vi "ProcessArray.vi"(4 "Plot Data":bool, 6 "Aquire Data":bool, 8 "File Path In":path, 11 "array in":sgl[][](array[numeric])) -> (0 "file path out":path, 1 "residue":dbl, 2 "intercept":dbl, 3 "Array out":T1(array[cluster]))   [LabVIEW 2019, in "SMU.lvclass"]
uses:
  SMU.lvclass
  <vilib>/Utility/file.llb/Write Delimited Spreadsheet (string).vi
  <vilib>/Utility/file.llb/Write Delimited Spreadsheet (DBL).vi
  <vilib>/Analysis/NI_AALPro.lvlib
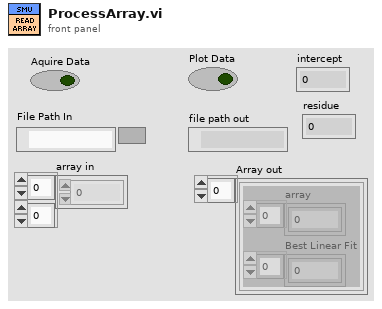
[diagram p1: front panel]
types:
  T1 = cluster{"array":sgl[], "Best Linear Fit":dbl[]}[]
  T2 = cluster{"array in":sgl[], "Best Linear Fit":dbl[]}
  T3 = cluster{"array in":sgl[], "Best Linear Fit":dbl[]}[]
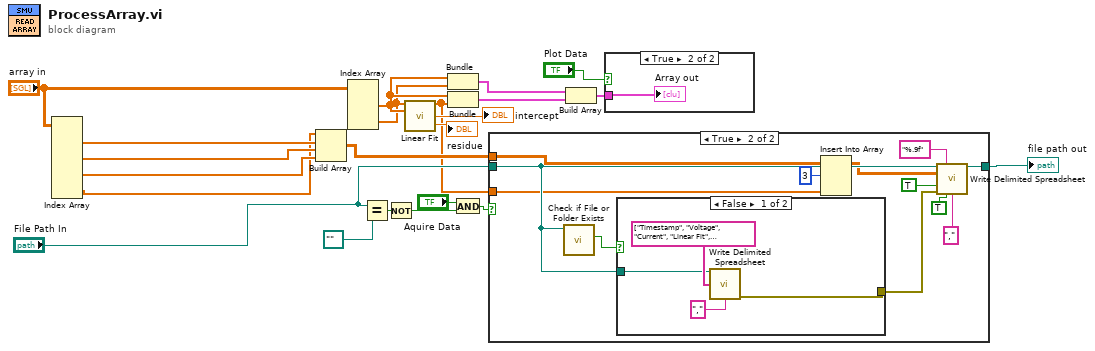
[diagram p0: block diagram]
diagram:
  n1 = Index Array(array="array in") -> (element #1=w6:sgl[], element #2=w2:sgl[], element #3=w5:sgl[], element #4=w1:sgl[])  [unwired: 8 in]
  n2 = Build Array(w1, w6, w2, w5) -> (w4:sgl[][])
  n3 = Index Array(array="array in") -> (element #1=w19:sgl[], element #2=w18:sgl[])  [unwired: 4 in]
  n4 = Equal?(x="File Path In", y=path "") -> (x = y?=w8:bool)
  n5 = Not(x=w8) -> (.not. x?=w20:bool)
  n6 = call <vilib>:"Linear Fit.vi"("Y"=w18, "X"=w19) -> ("Best Linear Fit"=w3:dbl[], "intercept"=→"intercept":dbl, "residue"=→"residue":dbl)  [unwired: 9 in, 2 out]
  n7 = Bundle("array in"=w19, "array in"=w18) -> (w16:cluster{"array in":sgl[], "array in":sgl[]})  [unwired: 1 in]
  n8 = Bundle("array in"=w19, "Best Linear Fit"=w3) -> (w17:T2)  [unwired: 1 in]
  n9 = And(x="Aquire Data", y=w20) -> (x .and. y?=w22:bool)
  n10 = case shown="True" w22 {
    tunnel: [w23 w35] -> w13
    tunnel: "File Path In" -> [w23 w31]
    tunnel: w4 -> [_ w28]
    tunnel: w3 -> [_ w25]
    frame False {
    }
    frame True {
      n11 = call <vilib>:"Check if File or Folder Exists.vi"("path"=w31) -> ("file or folder exists?"=w32:bool)  [unwired: 8 in, 2 out]
      n12 = case shown="False" w32 {
        tunnel: w31 -> [w38 _]
        tunnel: [w37 _] -> w30
        frame False {
          n13 = call-poly <vilib>:"Write Delimited Spreadsheet.vi"("file path (dialog if empty)"=w38, "1D data"=string[] ["Timestamp", "Voltage", "Current", "Linear Fit", "Resistance"], "delimiter (\\t)"="," ("delimiter (\\t)")) -> ("error out"=w37:errorcluster)  [unwired: 11 in, 1 out]
        }
        frame True {
        }
      }
      n14 = Insert Into Array(array=w28, index (row)=3, new element=w25) -> (w27:sgl[][])  [unwired: 1 in]
      n15 = call-poly <vilib>:"Write Delimited Spreadsheet.vi"("file path (dialog if empty)"=w31, "format (%.3f)"="%.9f" ("format (%s)"), "2D data"=w27, "append to file? (new file:F)"=TRUE, "error in (no error)"=w30, "transpose? (no:F)"=TRUE, "delimiter (\\t)"="," ("delimiter (\\t)")) -> ("new file path (Not A Path if cancelled)"=w35:path)  [unwired: 7 in, 1 out]
    }
  }
  "file path out" <- w13
  n16 = Build Array(w16, w17) -> (w15:T3)
  n17 = case shown="True" "Plot Data" {
    tunnel: w15 -> [_ w40]
    frame False {
    }
    frame True {
      "Array out" <- w40
    }
  }
